vi "sound files.vi"() -> ()   [LabVIEW 2020]
panel:
  in  "Start menu sound":path
  in  "Ladder up sound":path
  in  "Snake bite sound":path
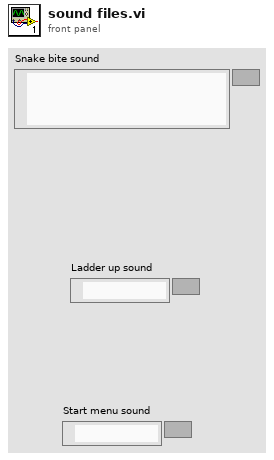
[diagram p1: front panel]
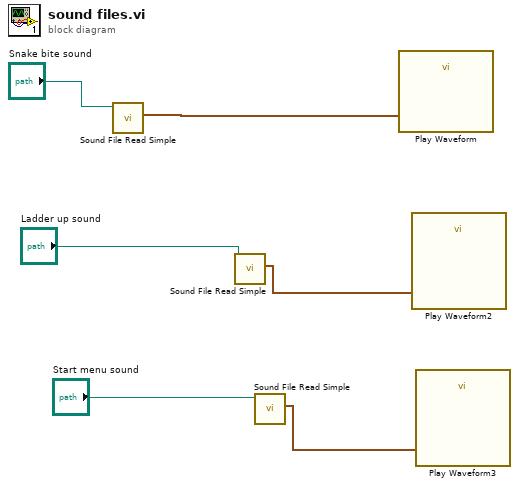
[diagram p0: block diagram]
diagram:
  n1 = call <vilib>:"Sound File Read Simple.vi"("path"="Snake bite sound") -> ("data"=w5:waveform(dbl)[])  [unwired: 7 in, 3 out]
  n2 = call <vilib>:"Sound File Read Simple.vi"("path"="Ladder up sound") -> ("data"=w3:waveform(dbl)[])  [unwired: 7 in, 3 out]
  n3 = call <vilib>:"Sound File Read Simple.vi"("path"="Start menu sound") -> ("data"=w4:waveform(dbl)[])  [unwired: 7 in, 3 out]
  n4 = call "Play Waveform"("Data"=w5) -> ()  [unwired: 18 in, 1 out]
  n5 = call "Play Waveform2"("Data"=w3) -> ()  [unwired: 18 in, 1 out]
  n6 = call "Play Waveform3"("Data"=w4) -> ()  [unwired: 18 in, 1 out]
